vi "Test Get VIs in project.vi"(8 "error in (no error)":errorcluster, 11 "Test Case In":refnum<class "Coverage Test.lvclass">) -> (0 "error out":errorcluster, 3 "Test Case Out":refnum<class "Coverage Test.lvclass">)   [LabVIEW 2020, in "LUnit Tests.lvlib" / "Coverage Test.lvclass"]
uses:
  Coverage Test.lvclass
  C:/Program Files (x86)/National Instruments/LabVIEW 2020/vi.lib/Astemes/LUnit/Test Case.lvclass
  source/Framework/Coverage Analyzer/Coverage Analyzer.lvclass
  <vilib>/Astemes/LUnit/Test Case.lvclass/Test Case.ctl
  <vilib>/Astemes/LUnit/LUnit Assertion Result.lvclass/LUnit Assertion Result.ctl
  <vilib>/Astemes/LUnit/LUnit Test Case Result.lvclass/LUnit Test Case Result.ctl
  <vilib>/Astemes/LUnit/LUnit Method Result.lvclass/LUnit Method Result.ctl
  b5a42e70-e756-42b2-85ed-2338bcd14d01.vi
  01074fa8-ee8a-411d-bc8b-fc92c4f90959.vi
  <vilib>/Astemes/LUnit/Palette/Pass.vi
  <vilib>/Astemes/LUnit/Palette/Fail.vi
  <vilib>/Astemes/LUnit/Compare Variants.vi
  <vilib>/Astemes/LUnit/Describe Comparison.vi
  <vilib>/Astemes/LUnit/Set Assertion Type.vi
  <vilib>/Astemes/LUnit/Add test result.vi
  <vilib>/Astemes/LUnit/LUnit Write Passed.vi
  <vilib>/Astemes/LUnit/LUnit Write Message.vi
  <vilib>/Astemes/LUnit/LUnit Write Description.vi
  <vilib>/Astemes/LUnit/Variant to string.vi
  <vilib>/Astemes/LUnit/LUnit Write Assertion Type.vi
  <vilib>/Astemes/LUnit/LUnit Record Assertion Result.vi
  <vilib>/Astemes/LUnit/LUnit Aggregate Assertion Results.vi
  <vilib>/Astemes/LUnit/Assertion Result/LUnit Read Status.vi
  <vilib>/Astemes/LUnit/LUnit Read Message.vi
  <vilib>/Astemes/LUnit/LUnit Read Description.vi
  <vilib>/Astemes/LUnit/Method Result/LUnit Merge Status.vi
  <vilib>/Astemes/LUnit/LUnit Concatenate result strings.vi
  <vilib>/Utility/Data Type/Get Type Information.vi
  <vilib>/Utility/LVClass/Get LV Class Name.vi
  <vilib>/Astemes/LUnit/LUnit Assertion Result.lvclass
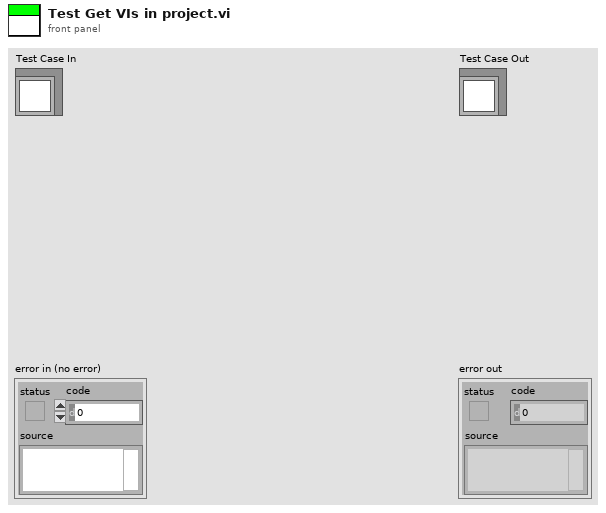
[diagram p1: front panel]
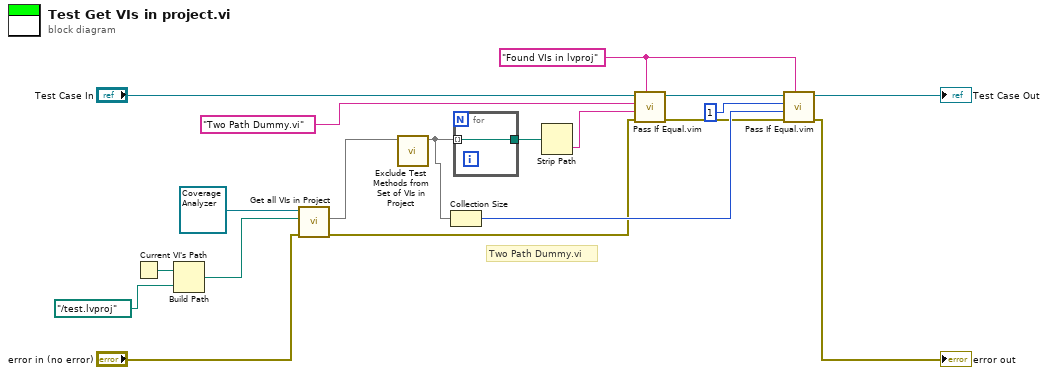
[diagram p0: block diagram]
diagram:
  w6 = "Found VIs in lvproj" ("Description")
  # "Two Path Dummy.vi"
  n1 = Current VI's Path() -> (path=w16:path)
  n2 = Build Path(base path=w16, name or relative path=path "../test.lvproj") -> (appended path=w14:path)
  n3 = call "Get all VIs in Project.vi"("error in (no error)"="error in (no error)", "Path"=w14, "Coverage Analyzer in"=refnum<class "Coverage Analyzer.lvclass"> refnum ("Coverage Analyzer.lvclass")) -> ("error out"=w10:errorcluster, "VIs"=w2:set{path})  [unwired: 6 in, 1 out]
  n4 = call "Exclude Test Methods from Set of VIs in Project.vi"("VIs"=w2) -> ("VIs 2"=w1:set{path})  [unwired: 10 in]
  n5 = Collection Size(1:w1) -> (0:w13:i32)
  n6 = for {
    tunnel: w1 -> [w20] mode=indexing
    tunnel: [w20] -> w5
  }
  n7 = Strip Path(path=w5) -> (name=w4:string)  [unwired: 1 out]
  n8 = call "Pass If Equal.vim"("Description"=w6, "error in (no error)"=w10, "Actual"=w4, "Expected"="Two Path Dummy.vi", "LUnit Test Case In"="Test Case In") -> ("error out"=w9:errorcluster, "LUnit Test Case Out"=w7:refnum<class "Coverage Test.lvclass">)  [unwired: 5 in]
  n9 = call "Pass If Equal.vim"("Description"=w6, "error in (no error)"=w9, "Actual"=w13, "Expected"=1 ("size(s)"), "LUnit Test Case In"=w7) -> ("error out"=→"error out":errorcluster, "LUnit Test Case Out"=→"Test Case Out":refnum<class "Coverage Test.lvclass">)  [unwired: 5 in]
